vi "Battery Identify First String.vi"(3 "ES String Data":T1) -> (1 "Index":i32)   [LabVIEW 2014]
uses:
  Controls/ES String Array.ctl
  Controls/ES String Data.ctl
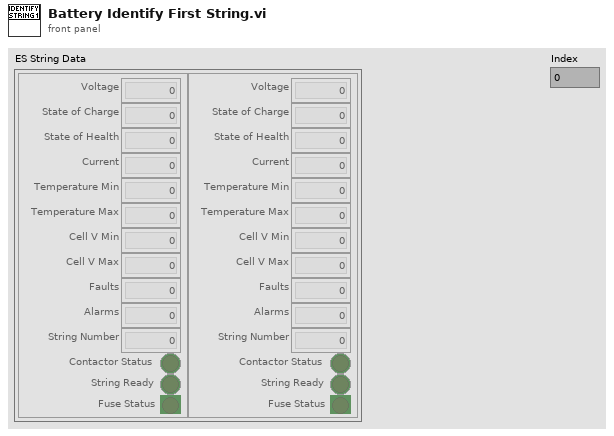
[diagram p1: front panel]
types:
  T1 = typedef "ES String Array.ctl" = T2[]
  T2 = typedef "ES String Data.ctl" = cluster{"Voltage":sgl, "State of Charge":sgl, "Current":sgl, "Temperature Min":i16, "Temperature Max":i16, "Faults":u16, "Alarms":u16, "String Number":u16, "Contactor Status":bool, "String Ready":bool, "Fuse Status":bool, "Cell V Max":dbl, "Cell V Min":dbl, "State of Health":sgl}
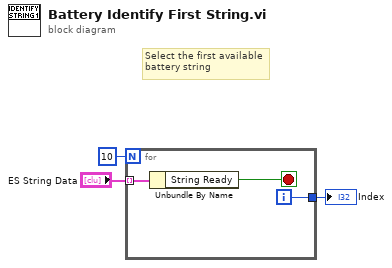
[diagram p0: block diagram]
diagram:
  # "Select the first available\nbattery string"
  n1 = for {
    N: 10 -> [_]
    tunnel: "ES String Data" -> [w6] mode=indexing
    tunnel: [w4] -> w1
    i -> [w4]
    stop <- w5 stop-if-true
    n2 = Unbundle By Name(w6) -> ("String Ready"=w5:bool)
  }
  "Index" <- w1
